vi "Set Delete If Outside Bounds.vi"(8 "Error In":errorcluster, 10 "Delete If Outside Bounds":bool, 11 "Display Element in":refnum<class "Display Element.lvclass">) -> (0 "Error Out":errorcluster, 3 "Display Element out":refnum<class "Display Element.lvclass">)   [LabVIEW 2019, in "Display Element.lvclass"]
uses:
  Display Element.lvclass
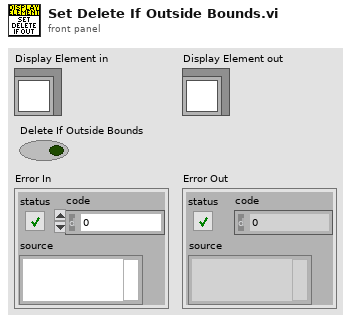
[diagram p1: front panel]
types:
  T1 = typedef "Display Element.lvclass/Data.ctl" = cluster{"Color":u32, "Layer":u32, "Tag":string, "Position":T2, "Force":T2, "Delete If Outside Bounds":bool}
  T2 = typedef "Display Element.lvclass/Vector.ctl" = cluster{"X":i32, "Y":i32}
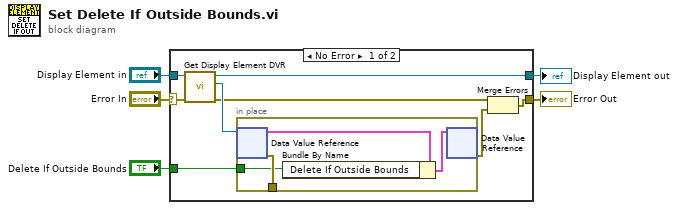
[diagram p0: block diagram]
diagram:
  n1 = case shown="No Error" "Error In" {
    selector: "Error In" -> [w10 w18]
    tunnel: [w12 w18] -> w4
    tunnel: [w8 w19] -> w2
    tunnel: "Display Element in" -> [w11 w19]
    tunnel: "Delete If Outside Bounds" -> [w6 _]
    frame No Error {
      n2 = call "Get Display Element DVR.vi"("Error In"=w10, "Display Element In"=w11) -> ("Error Out"=w7:errorcluster, "DVR"=w9:refnum<data-value>, "Display Element Out"=w8:refnum<class "Display Element.lvclass">)  [unwired: 7 in]
      n3 = in-place {
        in-place-border: [w17] -> _
        in-place-border: w6 -> [w14]
        n4 = in-place-dvr #1(w9) -> (w16:T1, w17:errorcluster)
        n5 = Bundle By Name(cluster=w16, "Delete If Outside Bounds"=w14) -> (w15:T1)
        n6 = in-place-dvr #1(w15) -> (w13:errorcluster)  [unwired: 1 out]
      }
      n7 = Merge Errors(w7, w13) -> (w12:errorcluster)
    }
    frame Error {
    }
  }
  "Display Element out" <- w2
  "Error Out" <- w4
